vi "SETPATHdll.vi"(8 "error in (no error)":errorcluster, 11 "hpath":string) -> (0 "error out":errorcluster, 2 "ln":i32, 3 "hpath out":string)   [LabVIEW 2016]
doc: "subroutine SETPATH (hpth, ln)\n\nset the path where the fluid files are located\n\nINPUTS:\nhpth -- location of the fluid files [character*255 variable]\n The path does not need to contain the ending \"\\\" and it can\n point directly to the location where the DLL is stored if a\n fluids subdirectory (with the corresponding fluid files) is\n located there.\n example: hpth='C:\\Program Files\\Refprop'\nhpth_length -- length of variable hpth (default: 255)"
uses:
  REFPROP.DLL
panel:
  # "REFPROP-SETPATHdll.vi"
  # "void  SETPATHdll(CStr hpath, int32_t ln)"
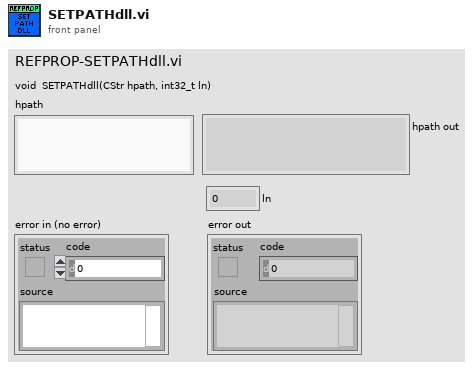
[diagram p1: front panel]
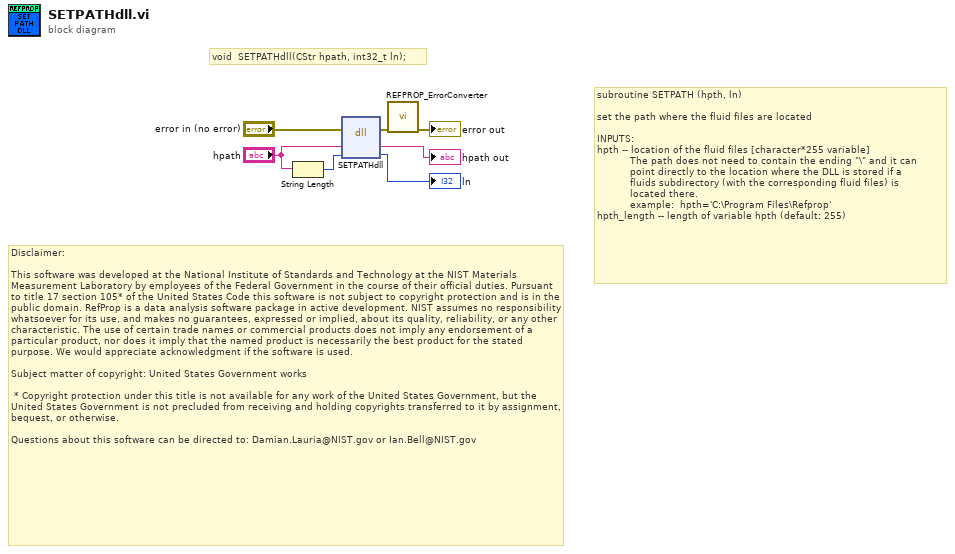
[diagram p0: block diagram]
diagram:
  # "Disclaimer:\n\nThis software was developed at the National Institute of Standards and Technology at the NIST Materials Measurement Laboratory by employees of the Federal Government in the course of their official duties. Pursuant to title 17 section 105* of the United States Code this software is not subject to copyright protection and is in the public domain. RefProp is a data analysis software package in active development. NIST assumes no responsibility whatsoever for its use, and makes no guarantees, expressed or implied, about its quality, reliability, or any other characteristic. The use of certain trade names or commercial products does not imply any endorsement of a particular product, nor does it imply that the named product is necessarily the best product for the stated purpose. We would appreciate acknowledgment if the software is used.\n \nSubject matter of copyright: United States Government works\n  \n * Copyright protection under this title is not available for any work of the United States Government, but the United States Government is not precluded from receiving and holding copyrights transferred to it by assignment, bequest, or otherwise.\n\nQuestions about this software can be directed to: Damian.Lauria@NIST.gov or Ian.Bell@NIST.gov"
  # "void  SETPATHdll(CStr hpath, int32_t ln);"
  # "subroutine SETPATH (hpth, ln)\n\nset the path where the fluid files are located\n\nINPUTS:\nhpth -- location of the fluid files [character*255 variable]\n           The path does not need to contain the ending \"\\\" and it can\n           point directly to the location where the DLL is stored if a\n           fluids subdirectory (with the corresponding fluid files) is\n           located there.\n           example:  hpth='C:\\Program Files\\Refprop'\nhpth_length -- length of variable hpth (default: 255)"
  n1 = String Length(string="hpath") -> (length=w3:i32)
  n2 = dll-call lib="S:/009 - Testing/02 - Performance Testing/REFPROP/REFPROP.*" fn="SETPATHdll"(error in="error in (no error)", "hpath"="hpath", "ln"=w3) -> (error out=w7:errorcluster, "hpath"=→"hpath out":string, "ln"=→"ln":i32)  [unwired: 3 in, 1 out]
  n3 = call "REFPROP_ErrorConverter.vi"("error in (no error)"=w7) -> ("error out"=→"error out":errorcluster)  [unwired: 10 in]
